vi "gRPC Client Cache FGV Impl.vi"(8 "error in":errorcluster, 9 "unique id in":u64, 10 "action":T3, 11 "vi references in":T1) -> (0 "error out":errorcluster, 1 "unique id out":u64, 2 "grpc client id":T2, 3 "cluster id":string)   [LabVIEW 2021, in "NI Discovery V1 Client.lvlib"]
uses:
  NI Discovery V1 Client.lvlib
  TypeDefs/gRPC Client Cache FGV Action.ctl
  <vilib>/gRPC/LabVIEW gRPC Library/Shared/grpcId.ctl
  TypeDefs/gRPC Client Cache VI References.ctl
  Measurements/Helpers/Error Strings Global Internal.vi
  <vilib>/gRPC/LabVIEW gRPC Library/grpc-lvsupport-release.lvlib
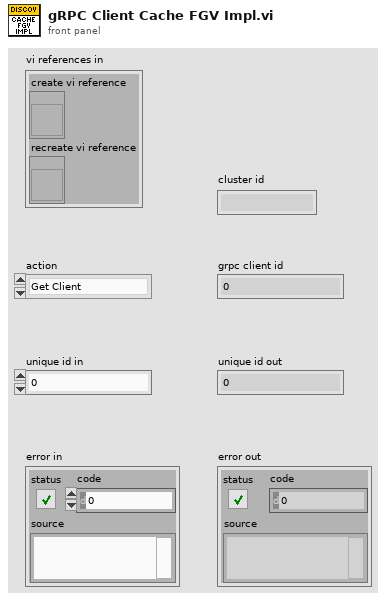
[diagram p1: front panel]
types:
  T1 = typedef "NI Discovery V1 Client.lvlib/gRPC Client Cache VI References.ctl" = cluster{"create vi reference":refnum<vi>, "recreate vi reference":refnum<vi>}
  T2 = typedef "grpc-lvsupport-release.lvlib/grpcId.ctl" = u64
  T3 = typedef "NI Discovery V1 Client.lvlib/gRPC Client Cache FGV Action.ctl" = enum16{"Get Client", "Recreate Client", "Destroy Client", "Update ClusterId"}
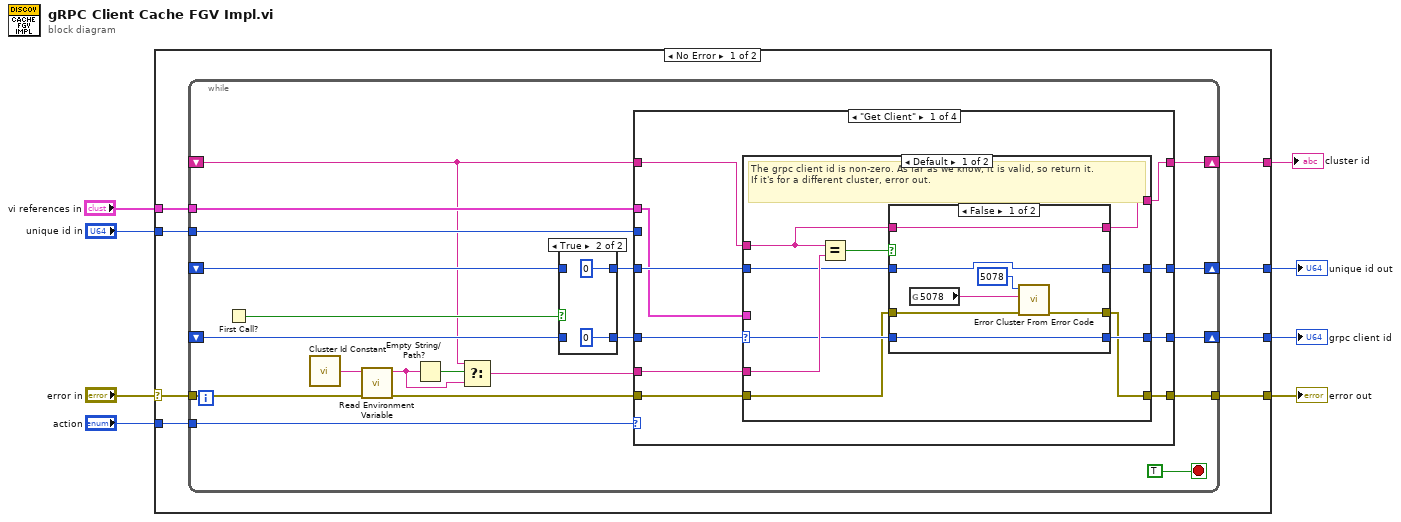
[diagram p0: block diagram]
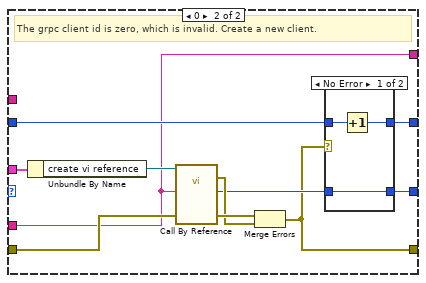
[diagram p4: hidden frame]
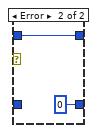
[diagram p5: hidden frame]
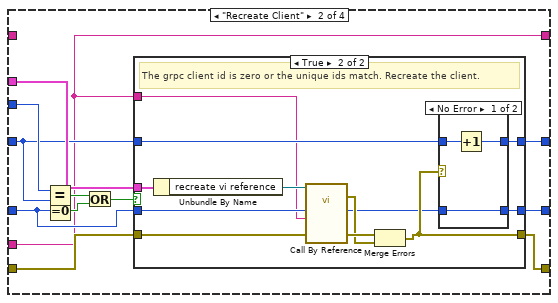
[diagram p6: hidden frame]
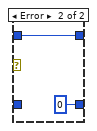
[diagram p8: hidden frame]
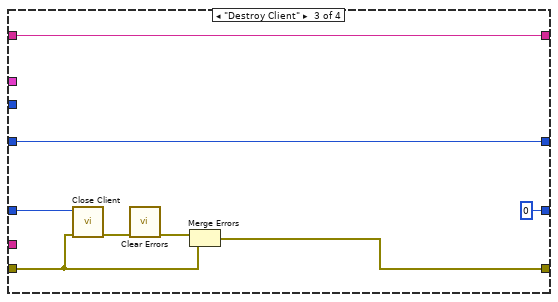
[diagram p9: hidden frame]
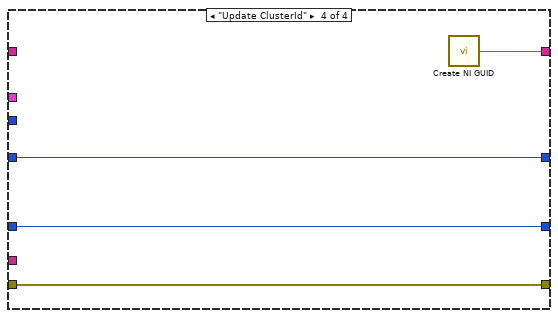
[diagram p10: hidden frame]
diagram:
  n1 = case shown="No Error" "error in" {
    selector: "error in" -> [w15 w132]
    tunnel: [w14 w132] -> w8
    tunnel: "action" -> [w16 _]
    tunnel: [w13 _] -> w7
    tunnel: [w12 _] -> w6
    tunnel: "unique id in" -> [w11 _]
    tunnel: "vi references in" -> [w10 _]
    tunnel: [w9 _] -> w1
    frame No Error {
      n2 = while {
        tunnel: w16 -> [w35]
        tunnel: w15 -> [w23]
        tunnel: [w34] -> w14
        shift-right: [w33] -> w13
        shift-left: _ -> [w31]
        shift-right: [w27] -> w12
        shift-left: _ -> [w29]
        tunnel: w11 -> [w26]
        tunnel: w10 -> [w25]
        shift-right: [w24] -> w9
        shift-left: _ -> [w20]
        stop <- TRUE stop-if-true
        n3 = First Call?() -> (First Call?: T/F=w32:bool)
        n4 = call "Cluster Id Constant.vi"() -> ("cluster id env"=w17:string)
        n5 = call "Read Environment Variable.vi"("error in"=w23, "name"=w17) -> ("error out"=w22:errorcluster, "value"=w19:string)  [unwired: 8 in]
        n6 = Empty String/Path?(string/path=w19) -> (empty?=w21:bool)
        n7 = Select(t=w20, s=w21, f=w19) -> (s? t:f=w18:string)
        n8 = case shown="True" w32 {
          tunnel: w31 -> [w38 _]
          tunnel: [w38 T2 0 ("gRPC ID out")] -> w30
          tunnel: w29 -> [w37 _]
          tunnel: [w37 u64 0] -> w28
          frame False {
          }
          frame True {
          }
        }
        n9 = case shown="\"Get Client\"" w35 {
          tunnel: w22 -> [w47 w98 w123 w128]
          tunnel: [w50 w99 w125 w128] -> w34
          tunnel: [w49 w96 T2 0 ("grpc client id out") w129] -> w33
          tunnel: w30 -> [w48 w89 w124 w129]
          tunnel: w28 -> [w46 w94 w121 w130]
          tunnel: [w45 w93 w121 w130] -> w27
          tunnel: w26 -> [_ w97 _ _]
          tunnel: w25 -> [w44 w95 _ _]
          tunnel: [w42 w88 w120 w131] -> w24
          tunnel: w20 -> [w41 _ w120 _]
          tunnel: w18 -> [w43 w88 _ _]
          frame "Get Client" {
            n10 = case shown="Default" w48 {
              selector: w48 -> [w56 _]
              tunnel: w47 -> [w54 w81]
              tunnel: [w53 w73] -> w50
              tunnel: [w55 w76] -> w49
              tunnel: w46 -> [w58 w75]
              tunnel: [w57 w74] -> w45
              tunnel: w44 -> [_ w80]
              tunnel: w43 -> [w59 w72]
              tunnel: [w51 w72] -> w42
              tunnel: w41 -> [w52 _]
              frame Default {
                # "The grpc client id is non-zero. As far as we know, it is valid, so return it.\nIf it's for a different cluster, error out."
                n11 = Equal?(x=w52, y=w59) -> (x = y?=w60:bool)
                n12 = case shown="False" w60 {
                  tunnel: w58 -> [w61 w71]
                  tunnel: [w61 w71] -> w57
                  tunnel: w56 -> [w62 w70]
                  tunnel: [w62 w70] -> w55
                  tunnel: w54 -> [w65 w69]
                  tunnel: [w64 w69] -> w53
                  tunnel: w52 -> [w63 w68]
                  tunnel: [w63 w68] -> w51
                  frame False {
                    n13 = global read "Error Strings Global Internal.vi" "5078"() -> (w67:string)
                    n14 = call <vilib>:"Error Cluster From Error Code.vi"("error in (no error)"=w65, "error message (\"\")"=w67, "error code (0)"=5078) -> ("error out"=w64:errorcluster)  [unwired: 6 in]
                  }
                  frame True {
                  }
                }
              }
              frame 0 {
                # "The grpc client id is zero, which is invalid. Create a new client."
                n15 = Unbundle By Name(w80) -> ("create vi reference"=w82:refnum<vi>)
                n16 = call-by-ref "?"(reference=w82, "error in"=w81, "cluster id"=w72) -> (error out=w78:errorcluster, 0:"error out"=w79:errorcluster, "grpc client id"=w77:T2)  [unwired: 9 in, 1 out]
                n17 = Merge Errors(w79, w78) -> (w73:errorcluster)
                n18 = case shown="No Error" w73 {
                  tunnel: w75 -> [w85 w86]
                  tunnel: [w84 w86] -> w74
                  tunnel: w77 -> [w83 _]
                  tunnel: [w83 T2 0 ("grpc client id out")] -> w76
                  frame No Error {
                    n19 = Increment(x=w85) -> (x+1=w84:u64)
                  }
                  frame Error {
                  }
                }
              }
            }
          }
          frame "Recreate Client" {
            n20 = Equal?(x=w97, y=w94) -> (x = y?=w92:bool)
            n21 = Equal To 0?(x=w89) -> (x = 0?=w90:bool)
            n22 = Or(x=w92, y=w90) -> (x .or. y?=w91:bool)
            n23 = case shown="True" w91 {
              tunnel: w89 -> [w101 w112]
              tunnel: [w102 w108] -> w99
              tunnel: w98 -> [w102 w111]
              tunnel: [w101 w104] -> w96
              tunnel: w95 -> [_ w114]
              tunnel: w94 -> [w100 w107]
              tunnel: [w100 w106] -> w93
              tunnel: w88 -> [_ w103]
              frame False {
                # "The grpc client id is non-zero and the unique ids don't match. The client has already been recreated, so just return it."
              }
              frame True {
                # "The grpc client id is zero or the unique ids match. Recreate the client."
                n24 = Unbundle By Name(w114) -> ("recreate vi reference"=w113:refnum<vi>)
                n25 = call-by-ref "?"(reference=w113, "error in"=w111, "cluster id"=w103, "grpc client id in"=w112) -> (error out=w109:errorcluster, 0:"error out"=w110:errorcluster, "grpc client id out"=w105:T2)  [unwired: 8 in, 1 out]
                n26 = Merge Errors(w110, w109) -> (w108:errorcluster)
                n27 = case shown="No Error" w108 {
                  tunnel: w107 -> [w117 w119]
                  tunnel: [w116 w119] -> w106
                  tunnel: w105 -> [w115 _]
                  tunnel: [w115 T2 0 ("grpc client id out")] -> w104
                  frame No Error {
                    n28 = Increment(x=w117) -> (x+1=w116:u64)
                  }
                  frame Error {
                  }
                }
              }
            }
          }
          frame "Destroy Client" {
            n29 = call <vilib>:"Close Client.vi"("error in"=w123, "ClientID in"=w124) -> ("error out"=w122:errorcluster)  [unwired: 9 in]
            n30 = call <vilib>:"Clear Errors.vi"("error in (no error)"=w122) -> ("error out"=w126:errorcluster)  [unwired: 5 in, 1 out]
            n31 = Merge Errors(w126, w123) -> (w125:errorcluster)
          }
          frame "Update ClusterId" {
            n32 = call <vilib>:"Create NI GUID.vi"() -> ("NI GUID"=w131:string)
          }
        }
      }
    }
    frame Error {
    }
  }
  "error out" <- w8
  "grpc client id" <- w7
  "unique id out" <- w6
  "cluster id" <- w1
